vi "Get Owning Custom Device.vi"(8 "error in":errorcluster, 11 "item":T1 format="%.0x") -> (0 "error out":errorcluster, 2 "owning custom device":T1 format="%.0x", 3 "item out":T1 format="%.0x")   [LabVIEW 2020, in "AIM MIL-STD-1553 Scripting.lvlib"]
doc: "Returns the <b>description</b> section of the specified custom device."
uses:
  AIM MIL-STD-1553 Scripting.lvlib
  <vilib>/NI VeriStand/Custom Device Tools/Custom Device Utility Library/Custom Device Utility Library.lvlib
  <vilib>/NI VeriStand/Custom Device Tools/Custom Device Utility Library/Search Direction.ctl
  Constants.vi
  <vilib>/NI VeriStand/Custom Device Tools/Custom Device Utility Library/NI VeriStand - Search for Item by GUID.vi
  <vilib>/NI VeriStand/Custom Device API/Custom Device Item Ref.ctl
  <vilib>/NI VeriStand/Custom Device API/Custom Device API.lvlib
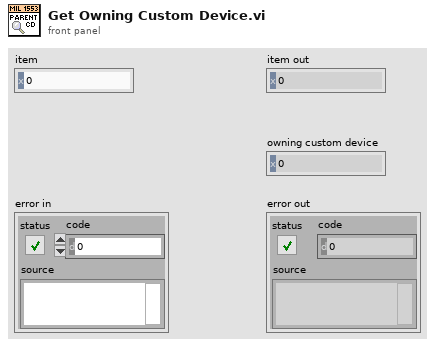
[diagram p1: front panel]
types:
  T1 = typedef "Custom Device API.lvlib/Custom Device Item Ref.ctl" = u64
  T2 = typedef "Custom Device Utility Library.lvlib/Search Direction.ctl" = enum16{"Down", "Up"}
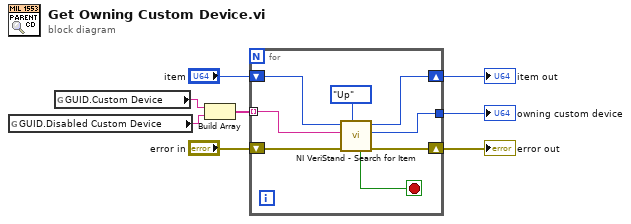
[diagram p0: block diagram]
diagram:
  n1 = global read "Constants.vi" "GUID.Disabled Custom Device"() -> (w2:string)
  n2 = global read "Constants.vi" "GUID.Custom Device"() -> (w3:string)
  n3 = Build Array(w3, w2) -> (w1:string[])
  n4 = for {
    tunnel: [w12] -> w4
    shift-right: [w14] -> w6
    shift-left: "error in" -> [w15]
    tunnel: w1 -> [w10] mode=indexing
    shift-right: [w13] -> w5
    shift-left: "item" -> [w16]
    stop <- w9 stop-if-true
    n5 = call-poly <vilib>:"NI VeriStand - Search for Item.vi"("Direction (Down)"=Search_Direction."Up", "error in"=w15, "Item GUID"=w10, "Section Ref in"=w16) -> ("error out"=w14:errorcluster, "Item Ref"=w12:T1, "Section Ref out"=w13:T1, "Found"=w9:bool)  [unwired: 4 in]
  }
  "item out" <- w5
  "error out" <- w6
  "owning custom device" <- w4
